vi "Display Info.vi"(7 "Layout ref":refnum<vi>, 8 "error in (no error)":errorcluster, 9 "Modify (F) /Add [T]":bool, 10 "Names in use":string[](array[string]), 11 "LTA-HS in":refnum<class "LTA-HS.lvclass">) -> (0 "error out":errorcluster, 1 "Names in use out":string[](array[string]), 2 "Changes Made?":bool, 3 "LTA-HS out":refnum<class "LTA-HS.lvclass">)   [LabVIEW 2013, in "LTA-HS.lvclass"]
uses:
  LTA-HS.lvclass
  TypeDefs/ColumnAppearCluster.ctl
  LTA-HS.lvclass/LTA-HS.ctl
  ColumnVIs/Column/Column.lvclass
panel:
  in  "Run Mode Appearance":T1={"Column Name"="Run Mode", "Width"=30, "Bkgd"=[16448250], "Text"=[0]}
  in  "Position Column Appearance":T1={"Column Name"="Position", "Width"=30, "Bkgd"=[16448250], "Text"=[0]}
  in  "Device Description":string
  in  "Hardware Settings":T2={"PB Trigger Line"=65535, "Serial Port"="ASRL21::INSTR"}
  in  "Name":string
  in  "Done":bool
  in  "Cancel":bool
  # "Serial Port should be formatted like:\nASRL##::INSTR"
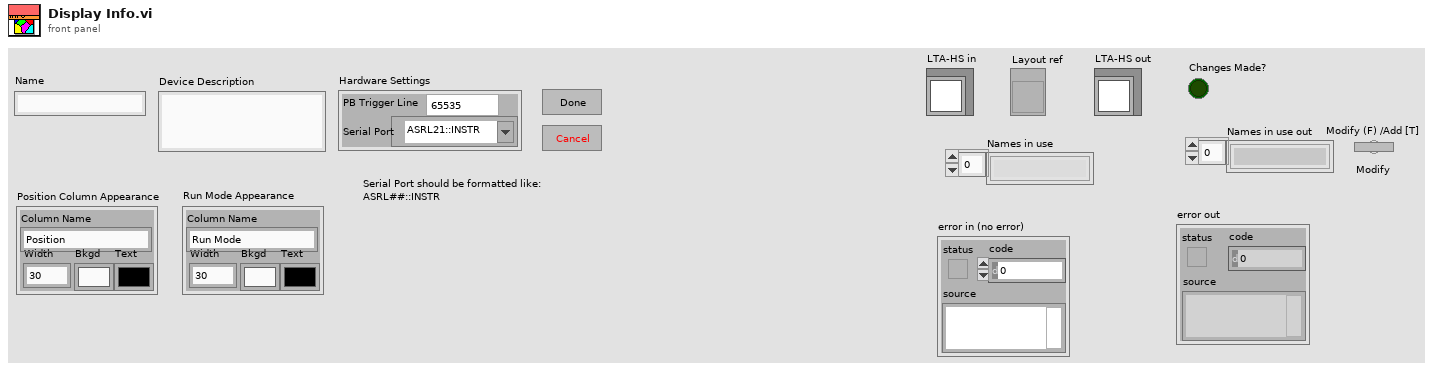
[diagram p1: front panel]
types:
  T1 = typedef "ColumnAppearCluster.ctl" = cluster{"Column Name":string, "Width":u32, "Bkgd":u32[], "Text":u32[]}
  T2 = cluster{"PB Trigger Line":u16, "Serial Port":refnum<visa-resource-name>}
  T3 = cluster{u16, "Serial Port":refnum<visa-resource-name>}
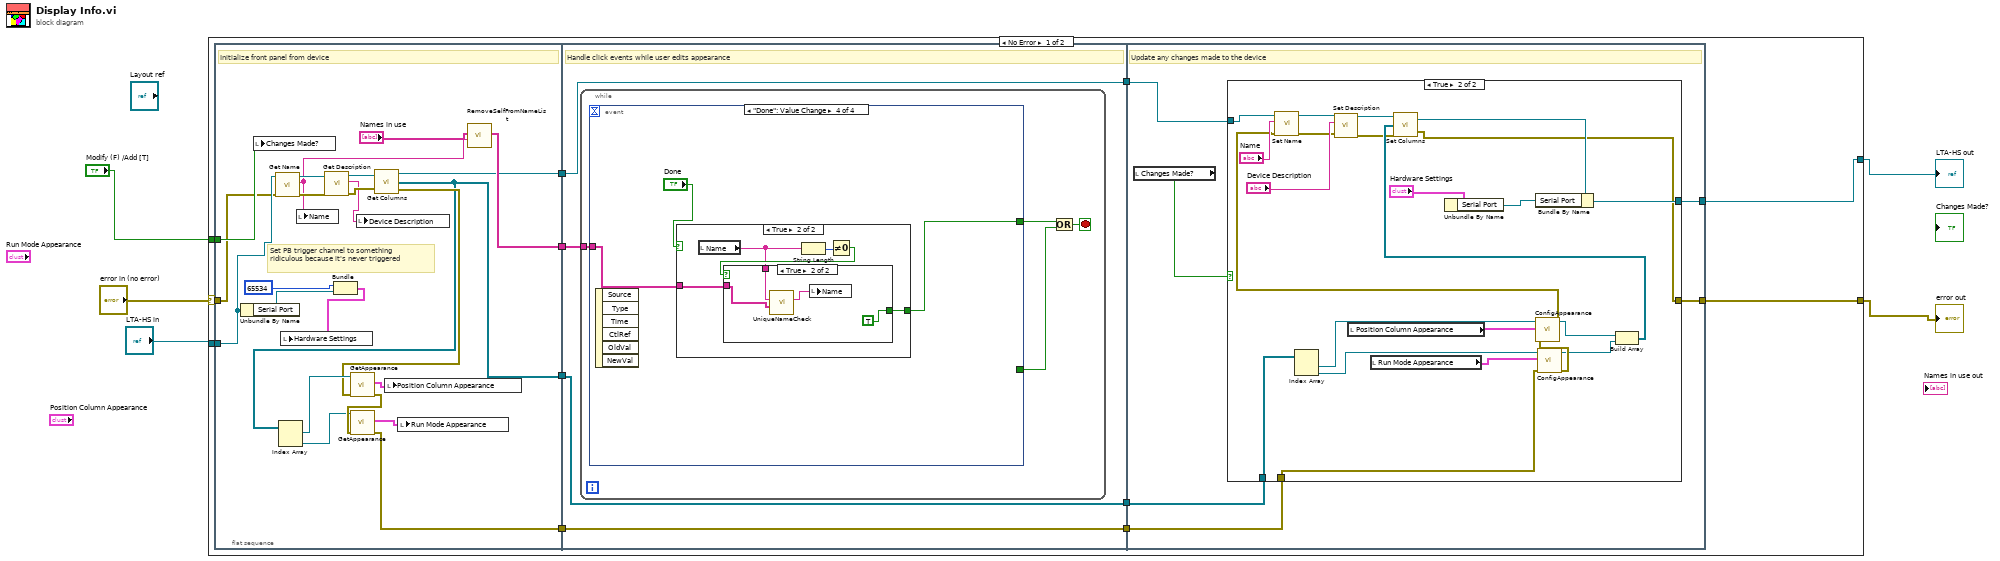
[diagram p0: block diagram]
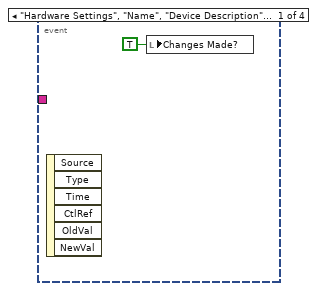
[diagram p2: hidden frame]
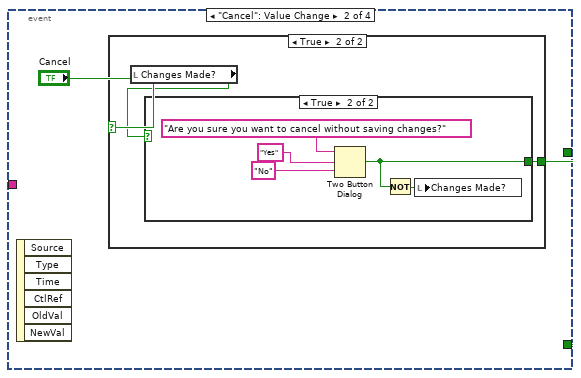
[diagram p3: hidden frame]
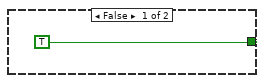
[diagram p5: hidden frame]
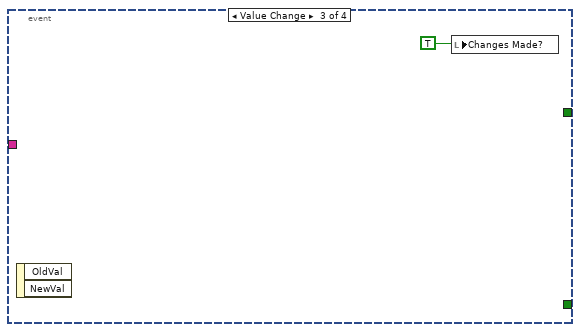
[diagram p6: hidden frame]
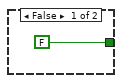
[diagram p7: hidden frame]
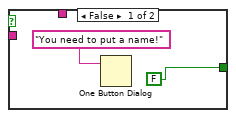
[diagram p8: hidden frame]
diagram:
  n1 = case shown="No Error" "error in (no error)" {
    selector: "error in (no error)" -> [w15 w109]
    tunnel: [w7 w109] -> w1
    tunnel: [w6 w108] -> w2
    tunnel: "LTA-HS in" -> [w16 w108]
    tunnel: "Modify (F) /Add [T]" -> [w17 _]
    frame No Error {
      n2 = flat-sequence {
        tunnel: w17 -> [w40]
        tunnel: w16 -> [w36]
        tunnel: w15 -> [w34]
        tunnel: [w25] -> w14
        tunnel: [w24] -> w13
        tunnel: [w23] -> w11
        tunnel: [w20] -> w9
        tunnel: w14 -> [w44]
        tunnel: w13 -> [w43]
        tunnel: [w43] -> w12
        tunnel: w11 -> [w42]
        tunnel: [w42] -> w10
        tunnel: w9 -> [w41]
        tunnel: [w41] -> w8
        tunnel: w12 -> [w82]
        tunnel: w10 -> [w81]
        tunnel: w8 -> [w80]
        tunnel: [w78] -> w7
        tunnel: [w77] -> w6
        frame #0 {
          # "Set PB trigger channel to something ridiculous because it's never triggered"
          # "Initialize front panel from device"
          n3 = Unbundle By Name(w36) -> ("Serial Port"=w38:refnum<visa-resource-name>)
          n4 = local write "Changes Made?"(w40) -> ()
          n5 = call-dynamic "Get Name.vi"("error in (no error)"=w34, "Device in"=w36) -> ("error out"=w33:errorcluster, "Name"=w30:string, "Device out"=w35:refnum<class "LTA-HS.lvclass">)  [unwired: 7 in]
          n6 = local write "Name"(w30) -> ()
          n7 = call-dynamic "Get Description.vi"("error in (no error)"=w33, "Device in"=w35) -> ("error out"=w31:errorcluster, "Device Description"=w29:string, "Device out"=w32:refnum<class "LTA-HS.lvclass">)  [unwired: 7 in]
          n8 = Bundle(u16 65534, "Serial Port"=w38) -> (w37:T3)  [unwired: 1 in]
          n9 = local write "Hardware Settings"(w37) -> ()
          n10 = local write "Device Description"(w29) -> ()
          n11 = call-dynamic "Get Columns.vi"("Device in"=w32, "error in (no error)"=w31) -> ("Device out"=w24:refnum<class "LTA-HS.lvclass">, "Columns"=w23:refnum<class "Column.lvclass">[], "error out"=w27:errorcluster)
          n12 = Index Array(array=w23) -> (element #1=w28:refnum<class "Column.lvclass">, element #2=w19:refnum<class "Column.lvclass">)  [unwired: 2 in]
          n13 = call "GetAppearance.vi"("error in (no error)"=w27, "Column in"=w28) -> ("error out"=w21:errorcluster, "Column Appearance"=w26:T1)  [unwired: 7 in, 1 out]
          n14 = call "GetAppearance.vi"("error in (no error)"=w21, "Column in"=w19) -> ("error out"=w20:errorcluster, "Column Appearance"=w18:T1)  [unwired: 7 in, 1 out]
          n15 = local write "Position Column Appearance"(w26) -> ()
          n16 = local write "Run Mode Appearance"(w18) -> ()
          n17 = call "RemoveSelfFromNameList.vi"("self Name"=w30, "Names in use"="Names in use") -> ("Reserved Names"=w25:string[])  [unwired: 9 in]
        }
        frame #1 {
          # "Handle click events while user edits appearance"
          n18 = while {
            tunnel: w44 -> [w45]
            stop <- w48 stop-if-true
            n19 = event shown="[3] \"Done\": Value Change" {
              selector: _ -> [_ _ _ _]
              dyn-events: _ -> [_ _ _ _]
              timeout: _ -> [_ _ _ _]
              tunnel: [_ w51 _ _] -> w47
              tunnel: [_ _ _ w64] -> w46
              tunnel: w45 -> [_ _ _ w62]
              event "Hardware Settings", "Name", "Device Description": Value Change {
                n20 = event-data() -> ()  [unwired: 1 in, 6 out]
                n21 = local write "Changes Made?"(TRUE ("Changes Made?")) -> ()
              }
              event "Cancel": Value Change {
                n22 = event-data() -> ()  [unwired: 1 in, 6 out]
                n23 = case shown="True" "Cancel" {
                  selector: "Cancel" -> [w52 _]
                  tunnel: [w52 w54] -> w51
                  frame False {
                  }
                  frame True {
                    n24 = local read "Changes Made?"() -> (w53:bool)
                    n25 = case shown="True" w53 {
                      tunnel: [TRUE w57] -> w54
                      frame False {
                      }
                      frame True {
                        n26 = Two Button Dialog(message="Are you sure you want to cancel without saving changes?", 1:"No", 2:"Yes") -> (T button?=w57:bool)
                        n27 = Not(x=w57) -> (.not. x?=w56:bool)
                        n28 = local write "Changes Made?"(w56) -> ()
                      }
                    }
                  }
                }
              }
              event Value Change {
                n29 = event-data() -> ()  [unwired: 1 in, 2 out]
                n30 = local write "Changes Made?"(TRUE) -> ()
              }
              event "Done": Value Change {
                n31 = event-data() -> ()  [unwired: 1 in, 6 out]
                n32 = case shown="True" "Done" {
                  tunnel: [FALSE w68] -> w64
                  tunnel: w62 -> [_ w67]
                  frame False {
                  }
                  frame True {
                    n33 = local read "Name"() -> (w66:string)
                    n34 = String Length(string=w66) -> (length=w70:i32)
                    n35 = Not Equal To 0?(x=w70) -> (x != 0?=w69:bool)
                    n36 = case shown="True" w69 {
                      tunnel: [FALSE TRUE] -> w68
                      tunnel: w67 -> [_ w75]
                      tunnel: w66 -> [_ w74]
                      frame False {
                        n37 = One Button Dialog(message="You need to put a name!") -> ()  [unwired: 1 in, 1 out]
                      }
                      frame True {
                        n38 = call "UniqueNameCheck.vi"("Names in use"=w75, "Device Name"=w74) -> ("Unique name"=w73:string)  [unwired: 8 in, 1 out]
                        n39 = local write "Name"(w73) -> ()
                      }
                    }
                  }
                }
              }
            }
            n40 = Or(x=w46, y=w47) -> (x .or. y?=w48:bool)
          }
        }
        frame #2 {
          # "Update any changes made to the device"
          n41 = local read "Changes Made?"() -> (w79:bool)
          n42 = case shown="True" w79 {
            tunnel: w82 -> [w84 w107]
            tunnel: w81 -> [_ w102]
            tunnel: w80 -> [w83 w89]
            tunnel: [w83 w90] -> w78
            tunnel: [w84 w92] -> w77
            frame False {
            }
            frame True {
              n43 = Index Array(array=w102) -> (element #1=w101:refnum<class "Column.lvclass">, element #2=w86:refnum<class "Column.lvclass">)  [unwired: 2 in]
              n44 = local read "Position Column Appearance"() -> (w98:T1)
              n45 = local read "Run Mode Appearance"() -> (w87:T1)
              n46 = Unbundle By Name("Hardware Settings") -> ("Serial Port"=w93:refnum<visa-resource-name>)
              n47 = call "ConfigAppearance.vi"("error in (no error)"=w89, "Column Appearance"=w87, "Column in"=w86) -> ("error out"=w88:errorcluster, "Column out"=w85:refnum<class "Column.lvclass">)  [unwired: 7 in]
              n48 = call "ConfigAppearance.vi"("error in (no error)"=w88, "Column Appearance"=w98, "Column in"=w101) -> ("error out"=w100:errorcluster, "Column out"=w97:refnum<class "Column.lvclass">)  [unwired: 7 in]
              n49 = call-dynamic "Set Name.vi"("error in (no error)"=w100, "Name"="Name", "Device in"=w107) -> ("error out"=w99:errorcluster, "Device out"=w105:refnum<class "LTA-HS.lvclass">)  [unwired: 7 in]
              n50 = call-dynamic "Set Description.vi"("error in (no error)"=w99, "Device Description"="Device Description", "Device in"=w105) -> ("error out"=w94:errorcluster, "Device out"=w95:refnum<class "LTA-HS.lvclass">)  [unwired: 7 in]
              n51 = Build Array(w97, w85) -> (w96:refnum<class "Column.lvclass">[])
              n52 = call-dynamic "Set Columns.vi"("error in (no error)"=w94, "Columns"=w96, "Device in"=w95) -> ("error out"=w90:errorcluster, "Device out"=w91:refnum<class "LTA-HS.lvclass">)  [unwired: 1 in]
              n53 = Bundle By Name(cluster=w91, "Serial Port"=w93) -> (w92:refnum<class "LTA-HS.lvclass">)
            }
          }
        }
      }
    }
    frame Error {
    }
  }
  "error out" <- w1
  "LTA-HS out" <- w2
